vi "get_roi_set_overlay.vi"(4 "Current ROI Tool in":u32(ring)=8 items=["Zoom Tool"=8, "Selection Tool"=0, "Pan Tool"=9, "Point Tool"=1, "Line Tool"=2, "Rectangle Tool"=3, "Rotated Rectangle Tool"=12, "Polyline Tool"=10, "Polygon Tool"=5, "Freehand Tool"=11, "Closed Freehand Tool"=6, "Ellipse Tool"=4, "Annulus Tool"=7], 6 "ROI in":T2, 8 "error in":errorcluster, 11 "Reference Image in":T3) -> (0 "error out":errorcluster, 1 "counter out":i32, 3 "Reference Image out":T3)   [LabVIEW 2010, in "TrajectoryMH100122AODRAPS.lvclass"]
uses:
  TrajectoryMH100122AODRAPS.lvclass
  <vilib>/vision/Image Controls.llb/IMAQ Image.ctl
panel:
  in  "Font, Size & Style":T1={"Desired Font (Application)"=enum."Application Font", "[User-specified Font]"={"Font Name"="", "Size"=12, "Strikeout?"=FALSE, "Italic?"=FALSE, "Underline?"=FALSE, "Outline?"=FALSE, "Shadow?"=FALSE, "Bold?"=FALSE, "Rotation Angle"=0.0}, "Horizontal Alignment"=0, "Vertical Alignment"=0} {"Horizontal Alignment" items=["Left", "Center", "Right"]; "Vertical Alignment" items=["Bottom", "Top", "Baseline"]}
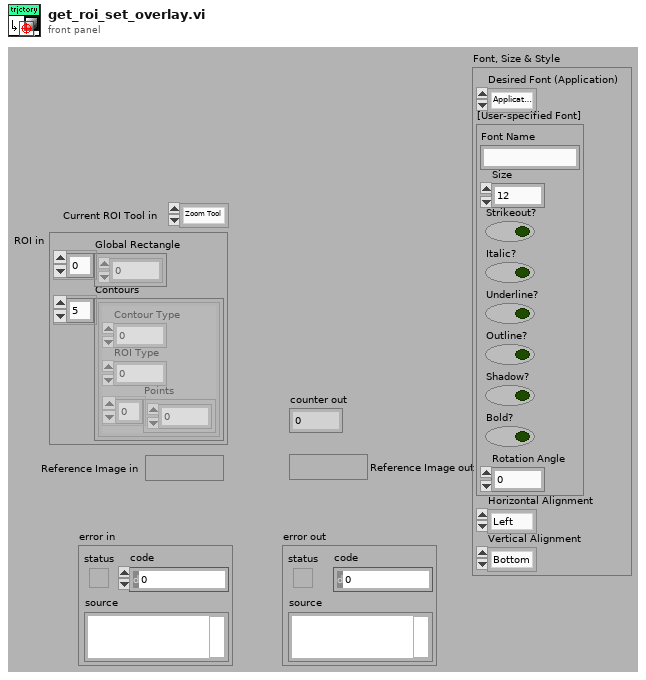
[diagram p1: front panel]
types:
  T1 = cluster{"Desired Font (Application)":enum16{"User-specified Font", "Application Font", "System Font", "Dialog Font"}, "[User-specified Font]":cluster{"Font Name":string, "Size":i16, "Strikeout?":bool, "Italic?":bool, "Underline?":bool, "Outline?":bool, "Shadow?":bool, "Bold?":bool, "Rotation Angle":dbl}, "Horizontal Alignment":i16, "Vertical Alignment":i16}
  T2 = cluster{"Global Rectangle":i32[], "Contours":cluster{"Contour Type":u32, "ROI Type":u32, "Points":i32[]}[]}
  T3 = typedef "IMAQ Image.ctl" = refnum<image>
  T4 = cluster{"Contour Type":u32, "ROI Type":u32, "Points":i32[]}[]
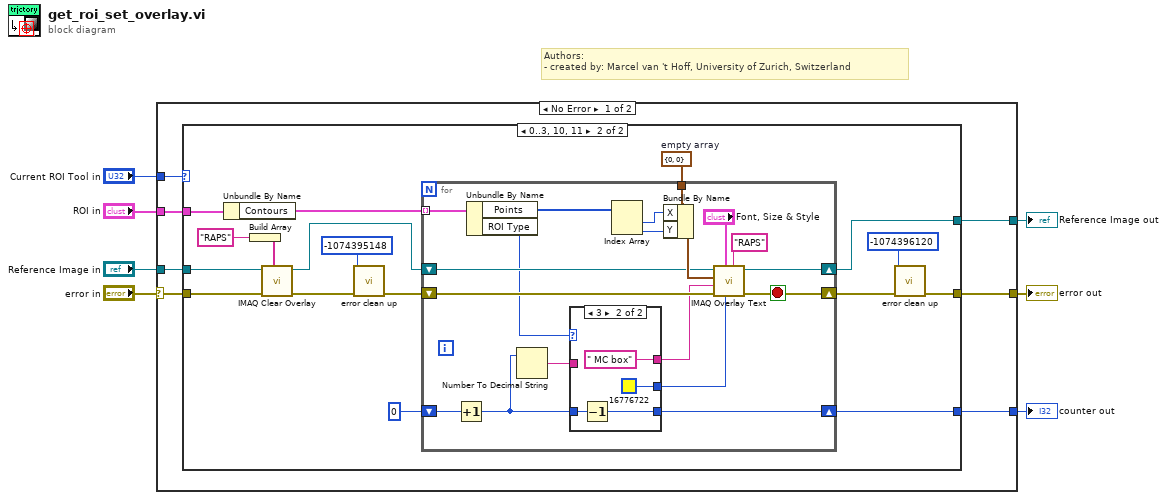
[diagram p0: block diagram]
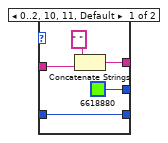
[diagram p3: hidden frame]
diagram:
  # "Authors: \n- created by: Marcel van 't Hoff, University of Zurich, Switzerland"
  n1 = case shown="No Error" "error in" {
    selector: "error in" -> [w12 w63]
    tunnel: [w14 w63] -> w7
    tunnel: "Reference Image in" -> [w13 w62]
    tunnel: [w11 w62] -> w4
    tunnel: "Current ROI Tool in" -> [w10 _]
    tunnel: "ROI in" -> [w9 _]
    tunnel: [w8 _] -> w1
    frame No Error {
      n2 = case shown="0..3, 10, 11" w10 {
        tunnel: [w15 w25] -> w14
        tunnel: w13 -> [w16 w31]
        tunnel: w12 -> [w15 w30]
        tunnel: [w16 w32] -> w11
        tunnel: w9 -> [_ w33]
        tunnel: [_ w24] -> w8
        frame Default {
        }
        frame 0..3, 10, 11 {
          w29 = cluster{"X":i32, "Y":i32} {"X"=0, "Y"=0}  # empty array
          n3 = Unbundle By Name(w33) -> ("Contours"=w28:T4)
          n4 = Build Array("RAPS" ("String")) -> (w23:string[])
          n5 = call "IMAQ Clear Overlay"("Groups"=w23, "error in (no error)"=w30, "Image"=w31) -> ("error out"=w20:errorcluster, "Image Out"=w18:T3)  [unwired: 7 in]
          n6 = call "error clean up.vi"("error in"=w20, "code in"=-1074395148 ("code")) -> ("error out"=w19:errorcluster)  [unwired: 9 in]
          n7 = for {
            tunnel: w28 -> [w52] mode=indexing
            tunnel: w29 -> [w48]
            shift-right: [w43] -> w26
            shift-left: w19 -> [w44]
            shift-right: [w45] -> w32
            shift-left: w18 -> [w46]
            shift-right: [w36] -> w24
            shift-left: 0 ("x+1") -> [w35]
            stop <- w43 stop-if-true
            n8 = Increment(x=w35) -> (x+1=w34:i32)
            n9 = Unbundle By Name(w52) -> ("Points"=w51:i32[], "ROI Type"=w41:u32)
            n10 = Number To Decimal String(number=w34) -> (decimal integer string=w40:string)  [unwired: 1 in]
            n11 = case shown="3" w41 {
              tunnel: w40 -> [w57 _]
              tunnel: [w55 " MC box" ("string")] -> w39
              tunnel: [u32 6618880 ("Text Color (black)") u32 16776722 ("Text Color (black)")] -> w38
              tunnel: [w53 w58] -> w36
              tunnel: w34 -> [w53 w59]
              frame 0..2, 10, 11, Default {
                n12 = Concatenate Strings(" " ("string"), w57) -> (w55:string)
              }
              frame 3 {
                n13 = Decrement(x=w59) -> (x-1=w58:i32)
              }
            }
            n14 = Index Array(array=w51) -> (element #1=w50:i32, element #2=w49:i32)  [unwired: 2 in]
            n15 = Bundle By Name(cluster=w48, "X"=w50, "Y"=w49) -> (w47:cluster{"X":i32, "Y":i32})
            n16 = call "IMAQ Overlay Text"("Group"="RAPS", "Text Color (black)"=w38, "Font, Size & Style"="Font, Size & Style", "error in (no error)"=w44, "String"=w39, "Origin"=w47, "Image"=w46) -> ("error out"=w43:errorcluster, "Image Out"=w45:T3)  [unwired: 3 in]
          }
          n17 = call "error clean up.vi"("error in"=w26, "code in"=-1074396120) -> ("error out"=w25:errorcluster)  [unwired: 9 in]
        }
      }
    }
    frame Error {
    }
  }
  "error out" <- w7
  "Reference Image out" <- w4
  "counter out" <- w1
